vi "uSubscriber Get uPolicy.vi"(8 "error in (no error)":errorcluster, 11 "uClient_Subscriber in":refnum<class "uClient_Subscriber.lvclass">) -> (0 "error out":errorcluster, 2 "uPolicy":refnum<class "uPolicy.lvclass">, 3 "uClient_Subscriber out":refnum<class "uClient_Subscriber.lvclass">)   [LabVIEW 2023, in "uFramework.lvlib" / "uClient_Subscriber.lvclass"]
uses:
  uClient_Subscriber.lvclass
  uPolicy/uPolicy.lvclass
  uClient_Subscriber.lvclass/uClient_Subscriber.ctl
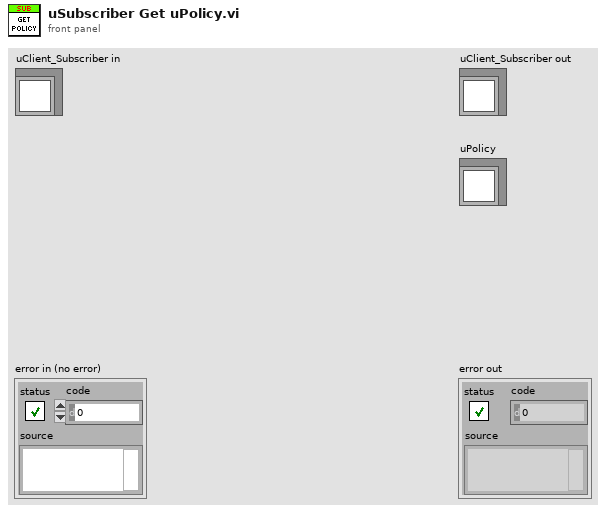
[diagram p1: front panel]
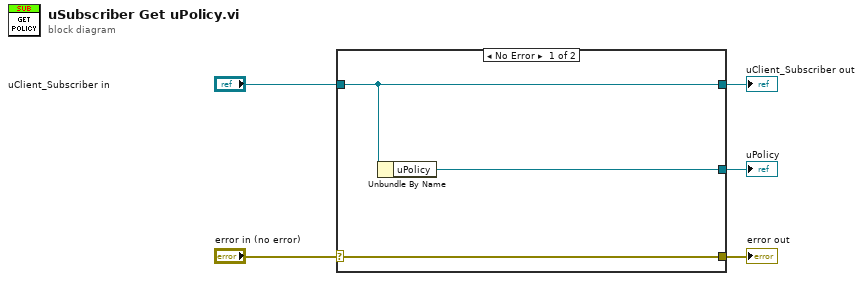
[diagram p0: block diagram]
diagram:
  n1 = case shown="No Error" "error in (no error)" {
    selector: "error in (no error)" -> [w8 w9]
    tunnel: [w8 w9] -> w4
    tunnel: [w7 w10] -> w2
    tunnel: "uClient_Subscriber in" -> [w7 w10]
    tunnel: [w6 _] -> w1
    frame No Error {
      n2 = Unbundle By Name(w7) -> ("uPolicy"=w6:refnum<class "uPolicy.lvclass">)
    }
    frame Error {
    }
  }
  "error out" <- w4
  "uClient_Subscriber out" <- w2
  "uPolicy" <- w1
